vi "Fetch (Output Buffer).vi"(8 "error in (no error)":errorcluster, 9 "Timeout (10000 ms)":u32=10000, 10 "Number of Samples (1)":i32=1, 11 "VISA resource name":refnum<visa-resource-name>) -> (0 "error out":errorcluster, 1 "End of Data?":bool, 2 "Measurements":dbl[](array[numeric]), 3 "VISA resource name out":refnum<visa-resource-name>)   [LabVIEW 2013, in "Agilent 34401.lvlib"]
doc: "This low level VI reads data from the output buffer and returns an array of values from the previously initiated measurement. The number of measurements the DMM takes is determined by the values you specify for the Trigger Count and Sample Count of the <B>Configure Multipoint VI</B>.\n\nThis VI is intended to be used in conjunction with the <B>Initiate (Output Buffer) VI</B>.\n\n<B>Note:</B>\n\n(1) This VI has been obsoleted from the driver and is included for compatibility with existing applications. New applications should use the <B>Fetch Measurement VI</B>.\n\n(2) This VI does not check the instrument status. Typically, you call this VI only in a sequence of calls to other low-level instrument driver VIs. The sequence performs one operation. You use the low-level VIs to optimize one or more aspects of interaction with the instrument. If you want to check the instrument status, call the <B>Error Query VI</B> at the conclusion of the sequence."
uses:
  <instrlib>/Agilent 34401/Agilent 34401.lvlib
panel:
  # "Note:\nThis VI has been obsoleted from the driver and is included for compatibility with existing applications.  New applications should use the Fetch Measurement VI."
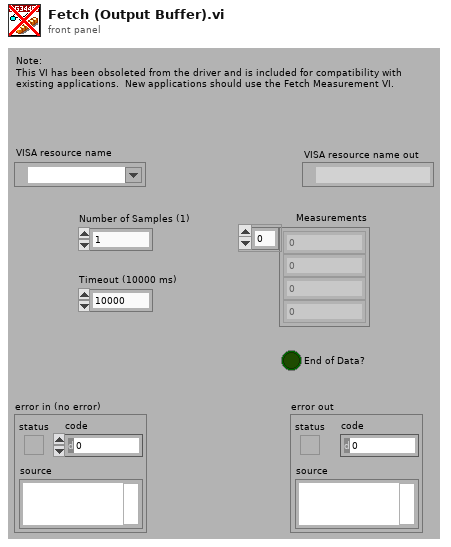
[diagram p1: front panel]
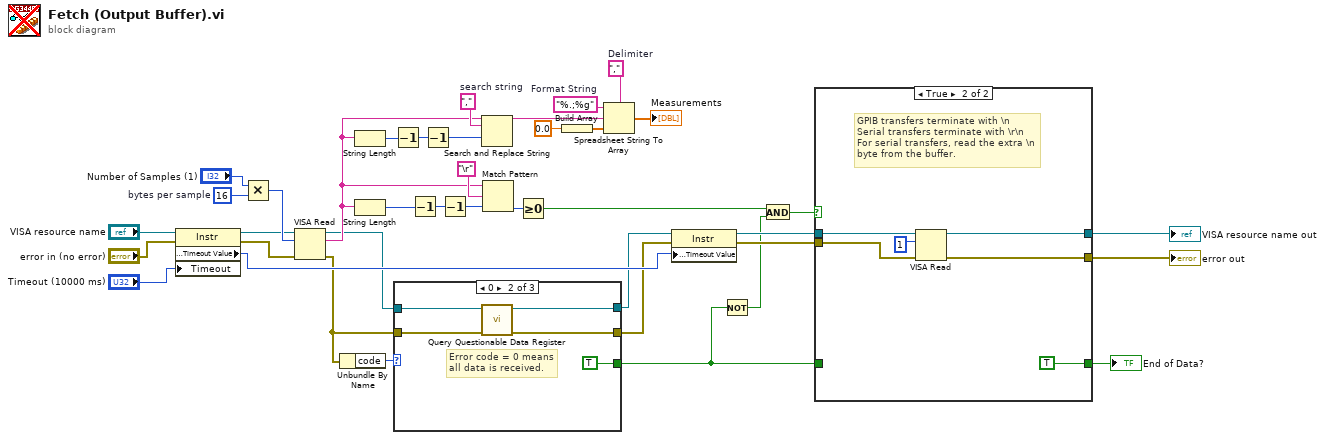
[diagram p0: block diagram]
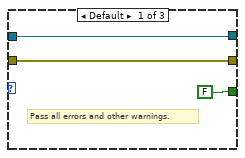
[diagram p2: hidden frame]
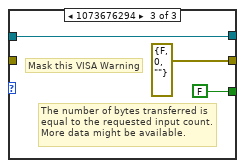
[diagram p3: hidden frame]
diagram:
  w25 = ","  # search string
  w35 = ","  # Delimiter
  w36 = "%.;%g"  # Format String
  w38 = u32 16  # bytes per sample
  n1 = property on="Property Node" class="Instr"(reference="VISA resource name", error in="error in (no error)", "Timeout"="Timeout (10000 ms)") -> (reference out=w29:refnum<visa-resource-name>, error out=w28:errorcluster, "General Settings:Timeout Value"=w27:u32)
  n2 = Multiply(x="Number of Samples (1)", y=w38) -> (x*y=w37:u32)
  n3 = VISA Read(VISA resource name=w29, byte count=w37, error in (no error)=w28) -> (VISA resource name out=w2:refnum<visa-resource-name>, read buffer=w15:string, error out=w11:errorcluster)  [unwired: 1 out]
  n4 = Unbundle By Name(w11) -> ("code"=w12:i32)
  n5 = String Length(string=w15) -> (length=w22:i32)
  n6 = String Length(string=w15) -> (length=w17:i32)
  n7 = Decrement(x=w22) -> (x-1=w23:i32)
  n8 = case shown="0" w12 {
    tunnel: w11 -> [w42 w46 _]
    tunnel: [w42 w44 errorcluster {"status"=FALSE, "code"=0, "source"=""} ("error out")] -> w10
    tunnel: [FALSE TRUE FALSE] -> w6
    tunnel: w2 -> [w40 w45 w48]
    tunnel: [w40 w43 w48] -> w1
    frame Default {
      # "Pass all errors and other warnings."
    }
    frame 0 {
      # "Error code = 0 means all data is received."
      n9 = call <instrlib>:"Query Questionable Data Register.vi"("error in (no error)"=w46, "VISA resource name"=w45) -> ("error out"=w44:errorcluster, "VISA resource name out"=w43:refnum<visa-resource-name>)  [unwired: 7 in, 1 out]
    }
    frame 1073676294 {
      # "Mask this VISA Warning"
      # "The number of bytes transferred is equal to the requested input count. More data might be available."
    }
  }
  n10 = Decrement(x=w17) -> (x-1=w18:i32)
  n11 = Decrement(x=w23) -> (x-1=w21:i32)
  n12 = Decrement(x=w18) -> (x-1=w16:i32)
  n13 = Search and Replace String(input string=w15, search string=w25, offset=w21) -> (result string=w24:string)  [unwired: 5 in, 3 out]
  n14 = Match Pattern(string=w15, regular expression="\r" ("Carriage Return Constant"), offset (0)=w16) -> (offset past match=w19:i32)  [unwired: 3 out]
  n15 = Greater Or Equal To 0?(x=w19) -> (x >= 0?=w8:bool)
  n16 = Build Array(0.0) -> (w33:dbl[])
  n17 = Spreadsheet String To Array(delimiter (Tab)=w35, format string=w36, spreadsheet string=w24, array type (2D Dbl)=w33) -> (array=→"Measurements":dbl[])
  n18 = property on="Property Node" class="Instr"(reference=w1, error in=w10, "General Settings:Timeout Value"=w27) -> (reference out=w14:refnum<visa-resource-name>, error out=w13:errorcluster)
  n19 = Not(x=w6) -> (.not. x?=w7:bool)
  n20 = And(x=w8, y=w7) -> (x .and. y?=w9:bool)
  n21 = case shown="True" w9 {
    tunnel: w14 -> [w53 w59]
    tunnel: w13 -> [w52 w58]
    tunnel: [w53 w56] -> w3
    tunnel: [w52 w54] -> w4
    tunnel: w6 -> [w51 _]
    tunnel: [w51 TRUE] -> w5
    frame False {
      # "For GPIB transfers, error condition, or incomplete serial operations, pass VISA session, error cluster and previously determined End of Data Boolean."
    }
    frame True {
      # "GPIB transfers terminate with \\n\nSerial transfers terminate with \\r\\n\nFor serial transfers, read the extra \\n byte from the buffer."
      n22 = VISA Read(VISA resource name=w59, byte count=u32 1, error in (no error)=w58) -> (VISA resource name out=w56:refnum<visa-resource-name>, error out=w54:errorcluster)  [unwired: 2 out]
    }
  }
  "VISA resource name out" <- w3
  "error out" <- w4
  "End of Data?" <- w5
